vi "command stack.vi"(7 "action":T1, 9 "selector":T2, 11 "command stack":T2[](array[typedef])) -> (1 "selector out":T2, 2 "stack is empty ?":bool, 3 "command stack out":T2[](array[typedef]))   [LabVIEW 2015]
uses:
  tale of three indices -- selector -- control.ctl
  stack action -- control.ctl
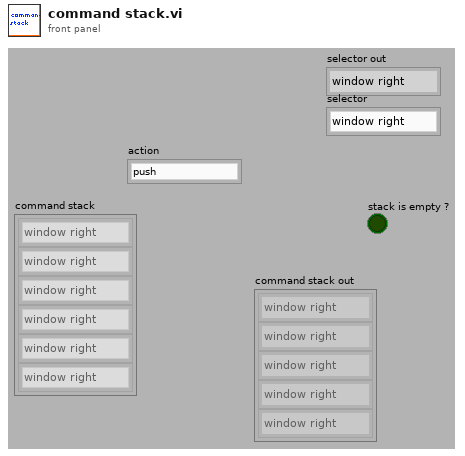
[diagram p1: front panel]
types:
  T1 = typedef "stack action -- control.ctl" = enum16{"push", "pop", "check", "init"}
  T2 = typedef "tale of three indices -- selector -- control.ctl" = enum16{"window right", "window left", "balance", "shrink", "grow", "do nothing", "reset", "center right", "center left", "all left", "all right", "right wing shrink", "left wing shrink", "left wing grow", "right wing grow", "skew left", "skew right", "check"}
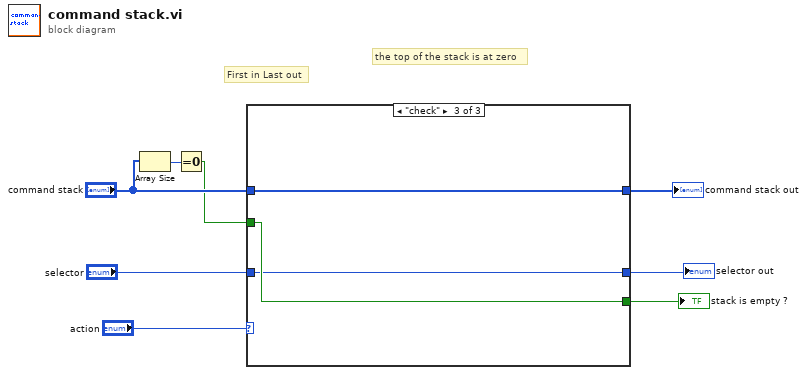
[diagram p0: block diagram]
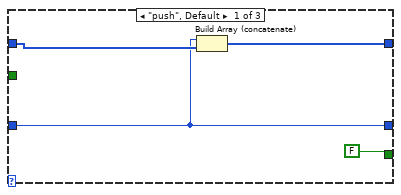
[diagram p2: hidden frame]
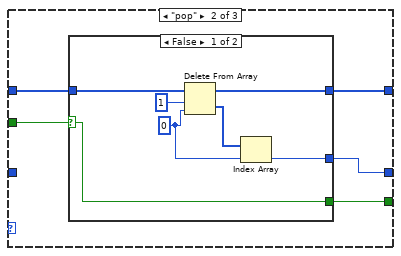
[diagram p3: hidden frame]
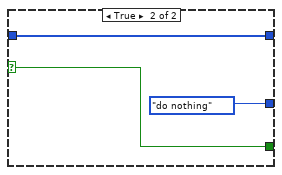
[diagram p4: hidden frame]
diagram:
  # "First in Last out"
  # "the top of the stack is at zero"
  n1 = Array Size(array="command stack") -> (size(s)=w6:i32)
  n2 = Equal To 0?(x=w6) -> (x = 0?=w5:bool)
  n3 = case shown="\"check\"" "action" {
    tunnel: [w11 w17 w28] -> w8
    tunnel: "command stack" -> [w12 w16 w28]
    tunnel: w5 -> [_ w15 w30]
    tunnel: [w10 w14 w29] -> w4
    tunnel: [FALSE w13 w30] -> w2
    tunnel: "selector" -> [w10 _ w29]
    frame "push", Default {
      n4 = Build Array (concatenate)(w10, w12) -> (w11:T2[])
    }
    frame "pop" {
      n5 = case shown="False" w15 {
        selector: w15 -> [w18 w25]
        tunnel: [w24 w27] -> w17
        tunnel: w16 -> [w23 w27]
        tunnel: [w19 tale_of_three_indices_--_selector_--_control."do nothing" ("selector out")] -> w14
        tunnel: [w18 w25] -> w13
        frame False {
          w20 = 0
          n6 = Delete From Array(array=w23, length=1, index=w20) -> (deleted portion=w21:T2[], array with subset deleted=w24:T2[])
          n7 = Index Array(array=w21, index=w20) -> (element=w19:T2)
        }
        frame True {
        }
      }
    }
    frame "check" {
    }
  }
  "command stack out" <- w8
  "stack is empty ?" <- w2
  "selector out" <- w4
